vi "Inicio Software.vi"() -> ()   [LabVIEW 2020]
panel:
  in  "ProgressBar":u8(slide) scale=0.0..100.0
  # "Control Versión 5.0\nSolicitado por: Dr. Gabriel Ramos Ortiz\nDesarrollo por: M.I. Enrique Noé Arias,\n                           M.O. Diego Torres Armenta"
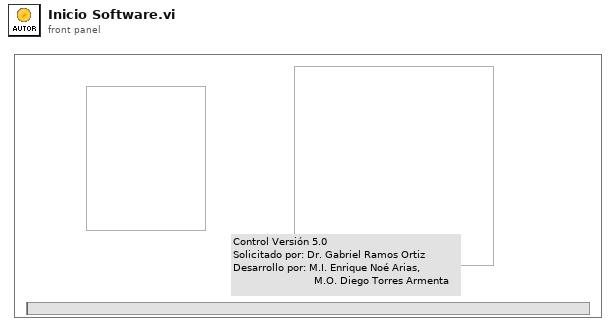
[diagram p1: front panel]
types:
  T1 = enum32{"Invalid", "Standard", "Closed", "Hidden", "Minimized", "Maximized"}
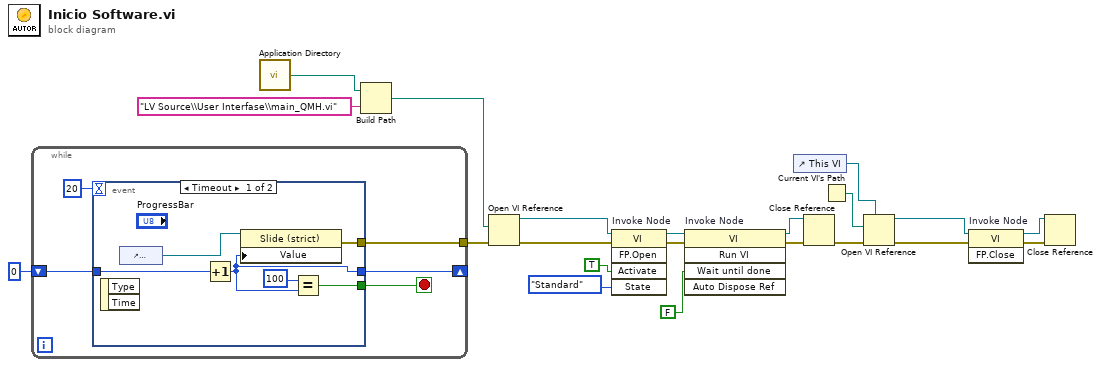
[diagram p0: block diagram]
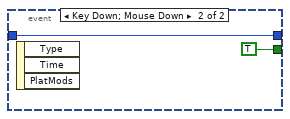
[diagram p2: hidden frame]
diagram:
  n1 = while {
    shift-right: [w23] -> _
    shift-left: u16 0 -> [w24]
    tunnel: [w22] -> w20
    stop <- w26 stop-if-true
    n2 = event shown="[0] Timeout" {
      selector: _ -> [_ _]
      dyn-events: _ -> [_ _]
      timeout: 20 -> [_ _]
      tunnel: [w31 TRUE] -> w26
      tunnel: w24 -> [w32 w33]
      tunnel: [w29 w33] -> w23
      tunnel: [w28 _] -> w22
      event Timeout {
        n3 = event-data() -> ()  [unwired: 1 in, 2 out]
        n4 = control-ref of="ProgressBar"() -> (w27:refnum<vi>)
        n5 = Increment(x=w32) -> (x+1=w29:u16)
        n6 = property class="Slide (strict)"(reference=w27, "Value"=w29) -> (error out=w28:errorcluster)  [unwired: 1 in, 1 out]
        n7 = Equal?(x=u16 100, y=w29) -> (x = y?=w31:bool)
      }
      event Key Down; Mouse Down {
        n8 = event-data() -> ()  [unwired: 1 in, 3 out]
      }
    }
  }
  n9 = call <vilib>:"Application Directory.vi"() -> ("Application Directory"=w3:path)
  n10 = Build Path(base path=w3, name or relative path="LV Source\\User Interfase\\main_QMH.vi") -> (appended path=w2:path)
  n11 = Open VI Reference(vi path=w2, error in (no error)=w20) -> (vi reference=w19:refnum<vi>, error out=w18:errorcluster)  [unwired: 4 in]
  n12 = invoke on="Invoke Node" class="VI" method="FP.Open"(reference=w19, error in=w18, "Activate"=TRUE ("Activate?"), "State"=T1."Standard") -> (reference out=w15:refnum<vi>, error out=w14:errorcluster)  [unwired: 1 in, 3 out]
  n13 = invoke on="Invoke Node" class="VI" method="Run VI"(reference=w15, error in=w14, "Wait until done"=FALSE ("Wait Until Done")) -> (reference out=w12:refnum<vi>, error out=w11:errorcluster)  [unwired: 2 in, 3 out]
  n14 = control-ref of="This VI"() -> (w4:refnum<vi>)
  n15 = Close Reference(reference=w12, error in (no error)=w11) -> (error out=w8:errorcluster)
  n16 = Current VI's Path() -> (path=w5:path)
  n17 = Open VI Reference(type specifier VI Refnum (for type only)=w4, vi path=w5, error in (no error)=w8) -> (vi reference=w10:refnum<vi>, error out=w9:errorcluster)  [unwired: 3 in]
  n18 = invoke on="Invoke Node" class="VI" method="FP.Close"(reference=w10, error in=w9) -> (reference out=w7:refnum<vi>, error out=w6:errorcluster)  [unwired: 1 in, 1 out]
  n19 = Close Reference(reference=w7, error in (no error)=w6) -> ()  [unwired: 1 out]
